vi "test-Ellip-Region-Constraint-Test2.vi"(8 "error in (no error)":errorcluster) -> (0 "error out":errorcluster, 3 "All tests passed":bool)   [LabVIEW 2019]
uses:
  <vilib>/Rock Robotics/WPI/ThirdParty/JAS_Junk/TrajLib/TypeDef/TRAJ_CONSTRAINT_ELLIP_REGION.ctl
  <vilib>/Rock Robotics/WPI/ThirdParty/JAS_Junk/TrajLib/TRANSLATION2D.ctl
  <vilib>/Rock Robotics/WPI/ThirdParty/JAS_Junk/TrajLib/Enum/TRAJ_CONSTRAINT_TYPES_ENUM.ctl
  <vilib>/Rock Robotics/WPI/ThirdParty/JAS_Junk/TrajLib/Rotation2d_CreateAngle.vi
  <vilib>/Rock Robotics/WPI/ThirdParty/JAS_Junk/TrajLib/VI/TrajConstraint_GetType.vi
  <vilib>/Rock Robotics/WPI/ThirdParty/JAS_Junk/TrajLib/Translation2d_RotateBy.vi
  <vilib>/Utility/Data Type/Get Type Information.vi
  <vilib>/Rock Robotics/WPI/ThirdParty/JAS_Junk/TrajLib/Trajectory_Library.lvlib
panel:
  out "Passed Test 2":bool
  out "Passed Test 1":bool
  out "ELLIP_REGION_CONSTRAINT":T1={"Center"={"X"=0.0, "Y"=0.0}, "Radii"={"X"=0.0, "Y"=0.0}, "Constraint"=variant, "Constraint Type"=enum."DIFF DRIVE KINEMATICS", "IM UNIQUE"=FALSE} {"Radii"."Y" format="%14.3f"; "Radii"."X" format="%14.3f"; "Center"."Y" format="%14.3f"; "Center"."X" format="%14.3f"}
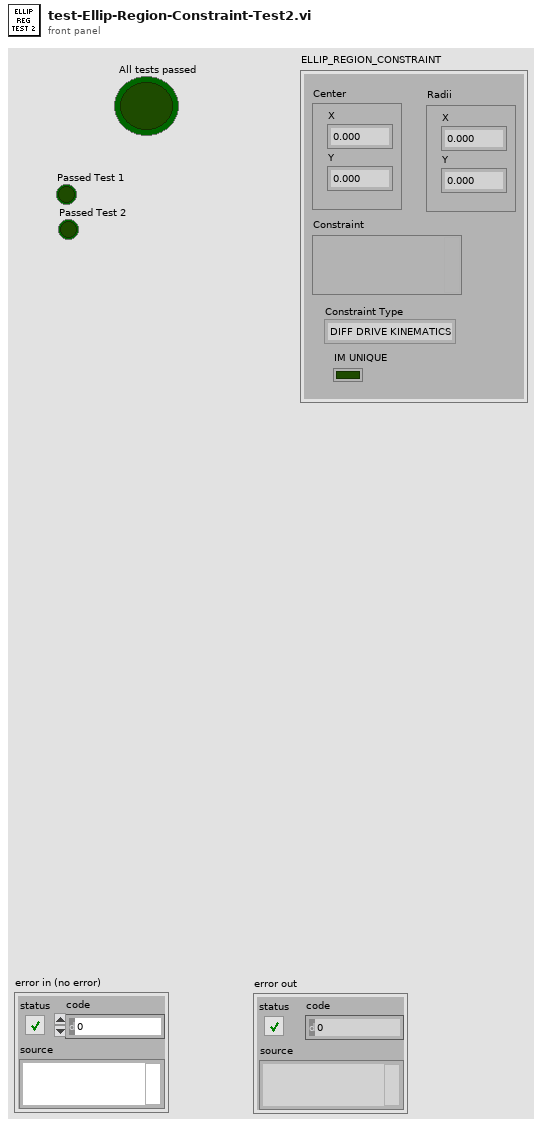
[diagram p1: front panel]
types:
  T1 = typedef "Trajectory_Library.lvlib/TRAJ_CONSTRAINT_ELLIP_REGION.ctl" = cluster{"Center":T2, "Radii":T2, "Constraint":variant, "Constraint Type":T3, "IM UNIQUE":bool}
  T2 = typedef "Trajectory_Library.lvlib/TRANSLATION2D.ctl" = cluster{"X":dbl, "Y":dbl}
  T3 = typedef "Trajectory_Library.lvlib/TRAJ_CONSTRAINT_TYPES_ENUM.ctl" = enum16{"UNDEFINED", "DIFF DRIVE KINEMATICS", "DIFF DRIVE VOLTAGE", "CENTRIPITAL ACCEL", "MECA DRIVE KINEMATICS", "SWERVE DRIVE KINEMATICS", "MAXIMUM VELOCITY", "ELLIPTICAL REGION", "RECTANGULAR REGION"}
  T4 = typedef "Trajectory_Library.lvlib/ROTATION2D.ctl" = cluster{"VALUE":dbl, "COS":dbl, "SIN":dbl}
  T5 = typedef "Trajectory_Library.lvlib/TRAJ_CONSTRAINT_MAX_VELOCITY.ctl" = cluster{"Max Velocity":dbl, "IM UNIQUE":bool}
  T6 = typedef "Trajectory_Library.lvlib/POSE2D.ctl" = cluster{"TRANSLATION":T2, "ROTATION":T4}
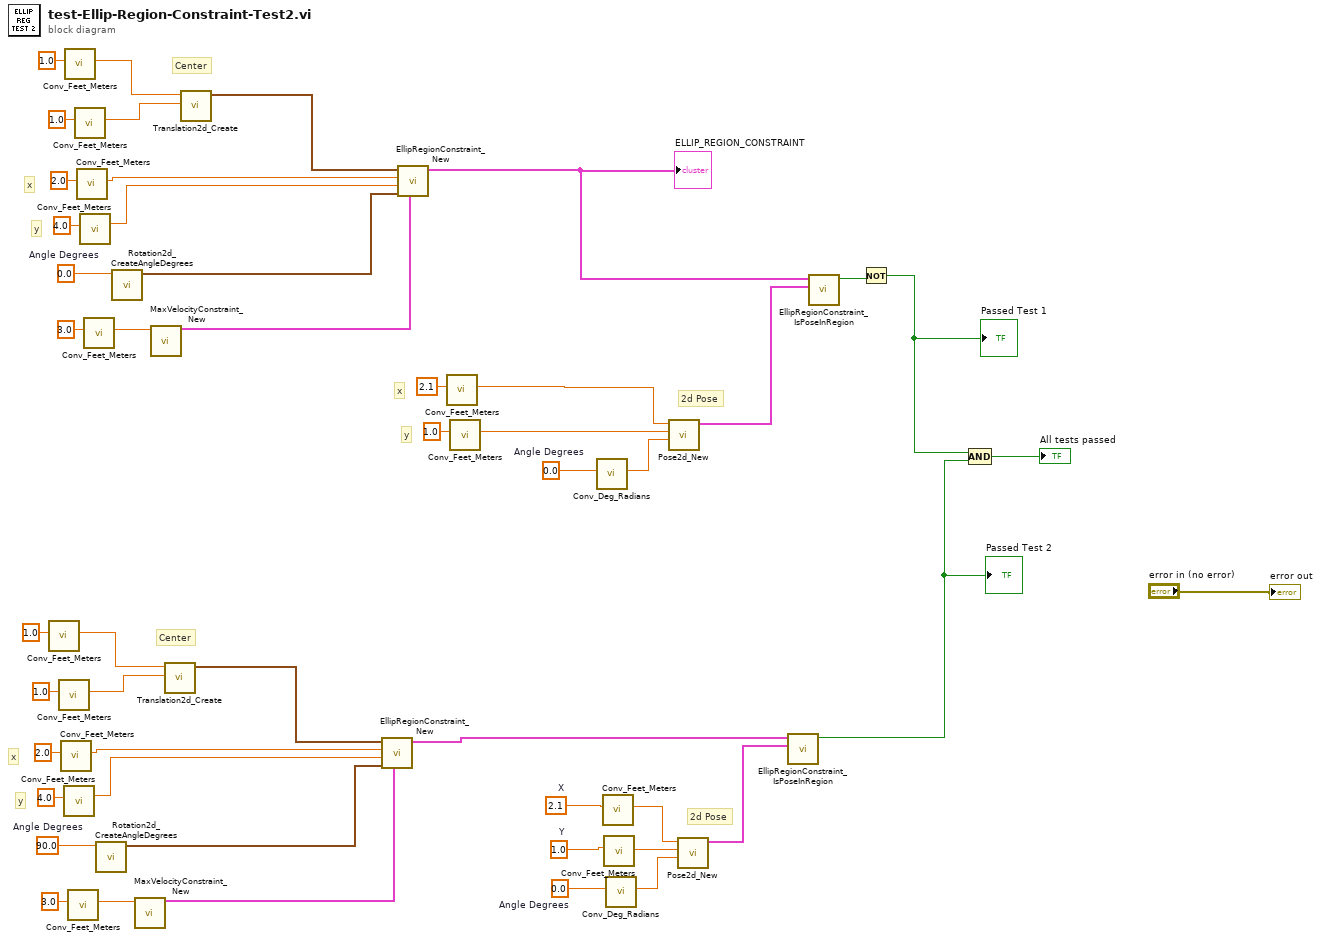
[diagram p0: block diagram]
diagram:
  w4 = 90.0  # Angle Degrees
  w23 = 0.0  # Angle Degrees
  w31 = 2.1  # X
  w30 = 1.0  # Y
  w33 = 0.0  # Angle Degrees
  w37 = 0.0  # Angle Degrees
  # "y"
  # "x"
  # "Center"
  # "y"
  # "x"
  # "y"
  # "x"
  # "2d Pose"
  # "2d Pose"
  # "Center"
  n1 = call <vilib>:"Conv_Feet_Meters.vi"("Feet"=1.0) -> ("Meters"=w10:dbl)  [unwired: 10 in]
  n2 = call <vilib>:"Conv_Feet_Meters.vi"("Feet"=1.0) -> ("Meters"=w9:dbl)  [unwired: 10 in]
  n3 = call <vilib>:"Conv_Feet_Meters.vi"("Feet"=2.0) -> ("Meters"=w6:dbl)  [unwired: 10 in]
  n4 = call <vilib>:"Conv_Feet_Meters.vi"("Feet"=4.0) -> ("Meters"=w5:dbl)  [unwired: 10 in]
  n5 = call <vilib>:"Conv_Feet_Meters.vi"("Feet"=1.0) -> ("Meters"=w42:dbl)  [unwired: 10 in]
  n6 = call <vilib>:"Conv_Feet_Meters.vi"("Feet"=3.0) -> ("Meters"=w8:dbl)  [unwired: 10 in]
  n7 = call <vilib>:"Conv_Feet_Meters.vi"("Feet"=1.0) -> ("Meters"=w41:dbl)  [unwired: 10 in]
  n8 = call <vilib>:"Conv_Feet_Meters.vi"("Feet"=2.0) -> ("Meters"=w25:dbl)  [unwired: 10 in]
  n9 = call <vilib>:"Conv_Feet_Meters.vi"("Feet"=4.0) -> ("Meters"=w24:dbl)  [unwired: 10 in]
  n10 = call <vilib>:"Conv_Feet_Meters.vi"("Feet"=3.0) -> ("Meters"=w40:dbl)  [unwired: 10 in]
  n11 = call <vilib>:"Rotation2d_CreateAngleDegrees.vi"("Angle_Degrees"=w4) -> ("ROTATION"=w3:T4)  [unwired: 10 in]
  n12 = call <vilib>:"Rotation2d_CreateAngleDegrees.vi"("Angle_Degrees"=w23) -> ("ROTATION"=w22:T4)  [unwired: 10 in]
  n13 = call <vilib>:"MaxVelocityConstraint_New.vi"("Maximum Velocity"=w8) -> ("MAX_VELOCITY_CONSTRAINT"=w7:T5)  [unwired: 10 in]
  n14 = call <vilib>:"MaxVelocityConstraint_New.vi"("Maximum Velocity"=w40) -> ("MAX_VELOCITY_CONSTRAINT"=w26:T5)  [unwired: 10 in]
  n15 = call <vilib>:"Translation2d_Create.vi"("Y"=w9, "X"=w10) -> ("TRANSLATION"=w15:T2)  [unwired: 9 in]
  n16 = call <vilib>:"Translation2d_Create.vi"("Y"=w41, "X"=w42) -> ("TRANSLATION"=w47:T2)  [unwired: 9 in]
  n17 = call <vilib>:"EllipRegionConstraint_New.vi"("Constraint Data Cluster"=w7, "Rotation"=w3, "Y Width"=w5, "X Width"=w6, "Center"=w15) -> ("ELLIP_REGION_CONSTRAINT"=w2:T1)  [unwired: 6 in]
  n18 = call <vilib>:"EllipRegionConstraint_New.vi"("Constraint Data Cluster"=w26, "Rotation"=w22, "Y Width"=w24, "X Width"=w25, "Center"=w47) -> ("ELLIP_REGION_CONSTRAINT"=w17:T1)  [unwired: 6 in]
  "ELLIP_REGION_CONSTRAINT" <- w17
  n19 = call <vilib>:"Conv_Feet_Meters.vi"("Feet"=2.1) -> ("Meters"=w19:dbl)  [unwired: 10 in]
  n20 = call <vilib>:"Conv_Feet_Meters.vi"("Feet"=1.0) -> ("Meters"=w18:dbl)  [unwired: 10 in]
  n21 = call <vilib>:"Conv_Deg_Radians.vi"("Degress"=w37) -> ("Radians"=w38:dbl)  [unwired: 10 in]
  n22 = call <vilib>:"Conv_Feet_Meters.vi"("Feet"=w31) -> ("Meters"=w29:dbl)  [unwired: 10 in]
  n23 = call <vilib>:"Conv_Feet_Meters.vi"("Feet"=w30) -> ("Meters"=w28:dbl)  [unwired: 10 in]
  n24 = call <vilib>:"Conv_Deg_Radians.vi"("Degress"=w33) -> ("Radians"=w34:dbl)  [unwired: 10 in]
  n25 = call <vilib>:"Pose2d_New.vi"("Heading"=w38, "Y"=w18, "X"=w19) -> ("out POSe"=w36:T6)  [unwired: 8 in]
  n26 = call <vilib>:"Pose2d_New.vi"("Heading"=w34, "Y"=w28, "X"=w29) -> ("out POSe"=w32:T6)  [unwired: 8 in]
  n27 = call <vilib>:"EllipRegionConstraint_IsPoseInRegion.vi"("statePose"=w32, "ELLIP_REGION_CONSTRAINT"=w2) -> ("PoseInRegion"=w1:bool)  [unwired: 9 in]
  "Passed Test 2" <- w1
  n28 = call <vilib>:"EllipRegionConstraint_IsPoseInRegion.vi"("statePose"=w36, "ELLIP_REGION_CONSTRAINT"=w17) -> ("PoseInRegion"=w35:bool)  [unwired: 9 in]
  n29 = Not(x=w35) -> (.not. x?=w27:bool)
  "Passed Test 1" <- w27
  n30 = Compound Arithmetic op=AND(w27, w1) -> (→"All tests passed":bool)
  "error out" <- "error in (no error)"
